vi "Bool_msg.vi"(11 "Boolean":bool) -> (3 "msg out":string)   [LabVIEW 2014]
uses:
  <vilib>/Tufts CEEO ROS for LabVIEW Software/ROS/MessageBuilding/std_msgs/subs/boolScalar.vi
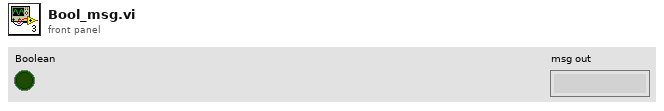
[diagram p1: front panel]
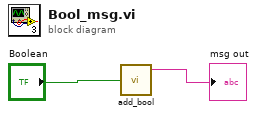
[diagram p0: block diagram]
diagram:
  n1 = call-poly <vilib>:"add_bool.vi"("Boolean"="Boolean") -> ("msg out"=→"msg out":string)  [unwired: 4 in]
